vi "myRIO_BRig_FPGA_v2,5__PortC.vi"() -> ()   [LabVIEW 2014]
uses:
  <vilib>/rvi/FXPMathLib/FxpDiv/subVIs/nifxpmath_Div_SimConfig.ctl
  <vilib>/rvi/FXPMathLib/FxpSinAndCos/subVIs/nifxpmath_SinAndCos_SimConfig.ctl
  <vilib>/rvi/FXPMathLib/FxpDiv/simVIs/DllFxpDivTemp_sub.vi
  <vilib>/rvi/FXPMathLib/FxpSinAndCos/simVIs/DllFxpSinAndCosTemp_sub.vi
  <vilib>/rvi/Emulation/niFpgaGetClockAttributes.vi
  <vilib>/rvi/Emulation/niFpgaSctlEmulationGetInTimedLoop.vi
  <vilib>/rvi/Emulation/niFpgaEmulationReportErrorSimple.vi
  <vilib>/rvi/eio/common/nirviEmuTemplateMethod_errors.vi
  <vilib>/rvi/Emulation/niFpgaCriticalErrorInLSC.vi
  <vilib>/rvi/FXPMathLib/FxpDiv/XNode/nifxpmath_Div.xnode
  <vilib>/rvi/FXPMathLib/FxpMul/XNode/nifxpmath_Multiplier.xnode
  <vilib>/rvi/FXPMathLib/FxpSinAndCos/XNode/nifxpmath_SinAndCos.xnode
  <vilib>/rvi/FXPMathLib/FxpSub/XNode/nifxpmath_Sub.xnode
  <vilib>/eio/EIONode/EIONode.xnode
  <vilib>/rvi/FXPMathLib/sim/FxpSim.dll
panel:
  in  "laserledMTrig":bool
  in  "tCycle_laser_wro":u32=100
  in  "tDelay_laser_wro":u32
  in  "tCycle_laser_rew":u32=100
  in  "tDelay_laser_rew":u32
  in  "laserResponse_reward_LED":bool
  in  "laserResponse_wrong_LED":bool
  out "SelectWrong":bool
  out "SelectReward":bool
  in  "laserResponse_wrong":bool
  in  "laserResponse_reward":bool
  in  "Left(F)_or_Right(T)":bool
  in  "ignoreWrong":bool
  in  "SelectionState":bool
  in  "laserMTrig":bool
  in  "FPGA_Stop":bool
  in  "audioTrigger_L":bool
  in  "audioTrigger_R":bool
  in  "audioFreq_L_Hz":u16=1000 min=1000 max=14000 step=1000
  in  "audioAmp_L":u16=1 min=1 max=32767 step=1
  in  "audioFreq_R_Hz":u16=1000 min=1000 max=14000 step=1000
  in  "audioAmp_R":u16=1 min=1 max=32767 step=1
  in  "A3_SL":bool
  in  "A1_SR":bool
  in  "Counts_Reset":bool
  out "A4_LickR":u32
  out "A2_LickL":u32
  in  "A6_Act":bool
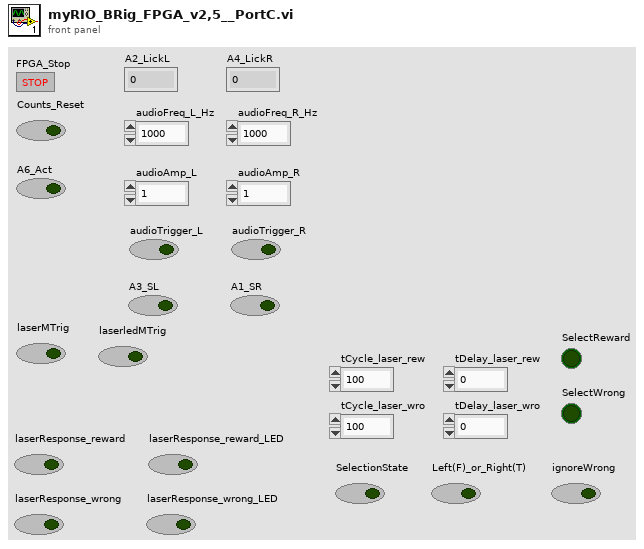
[diagram p1: front panel]
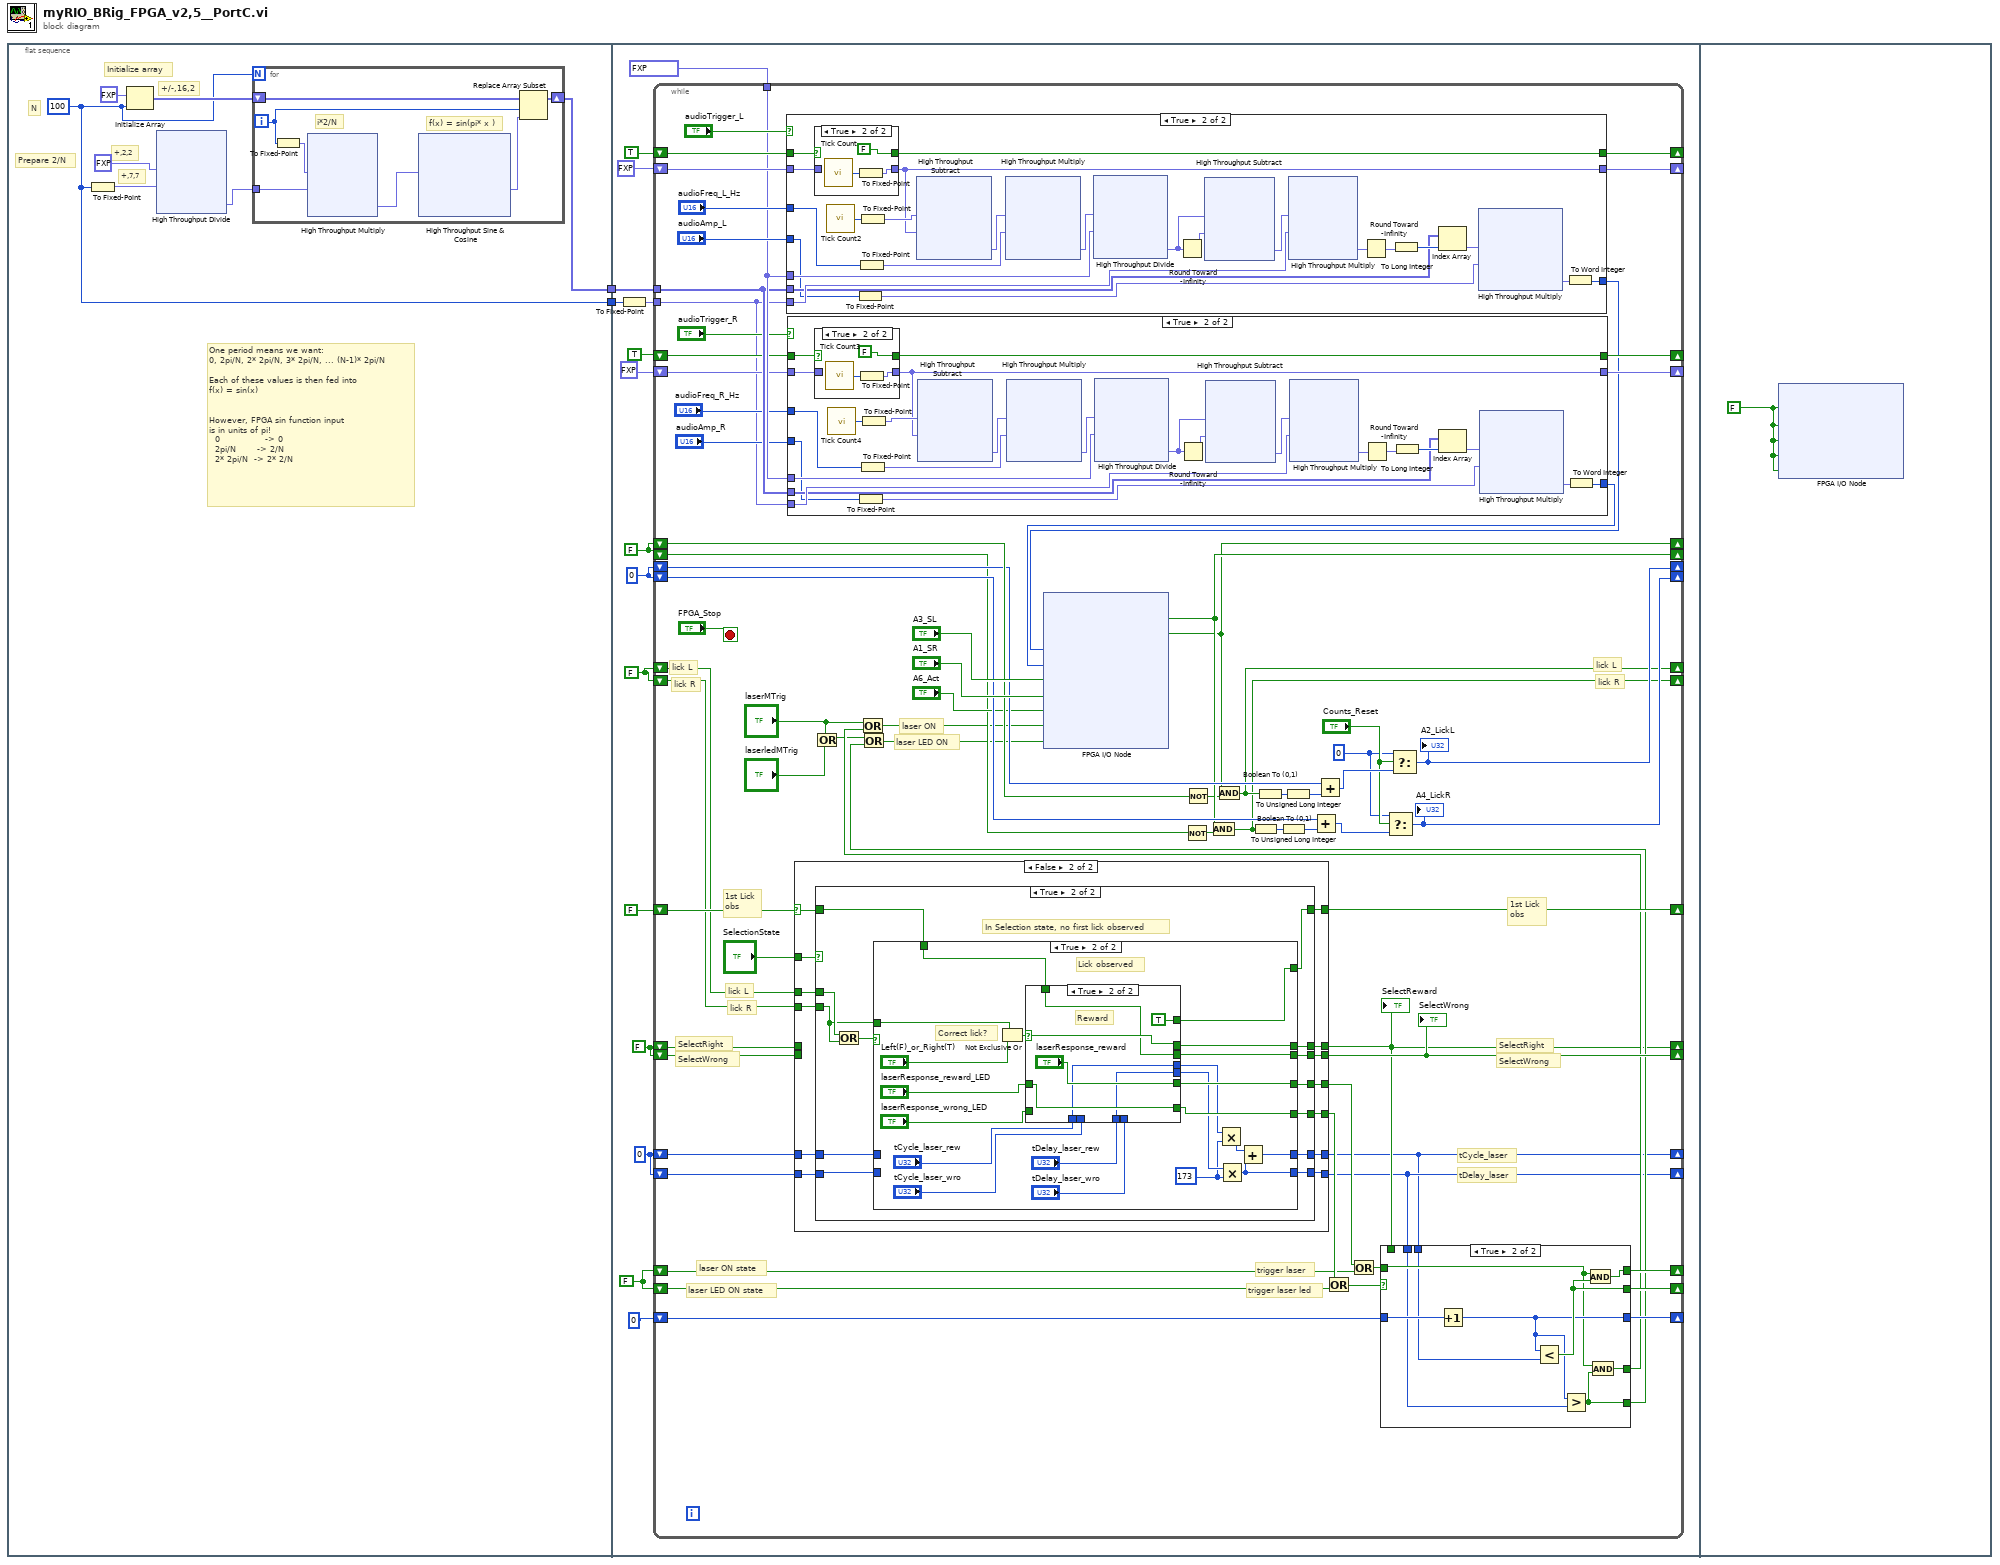
[diagram p0: block diagram]
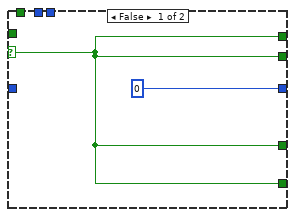
[diagram p2: hidden frame]
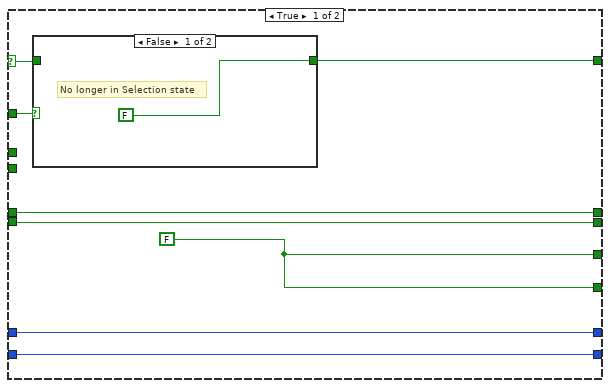
[diagram p3: hidden frame]
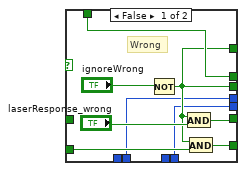
[diagram p7: hidden frame]
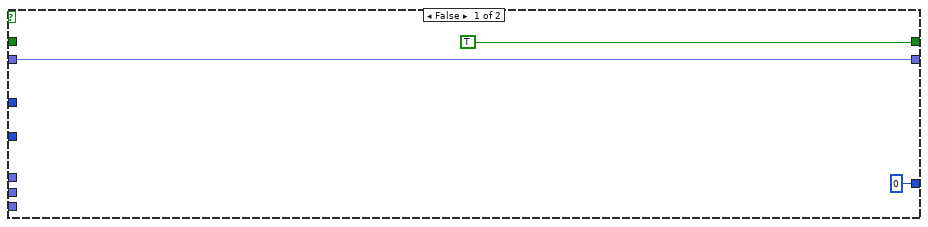
[diagram p8: hidden frame]
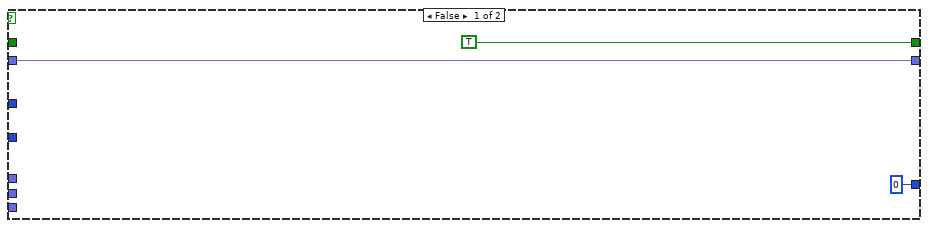
[diagram p10: hidden frame]
diagram:
  n1 = flat-sequence {
    tunnel: [w4] -> w2
    tunnel: [w3] -> w1
    tunnel: w2 -> [w84]
    tunnel: w1 -> [w86]
    frame #0 {
      w3 = 100 ("dimension size")
      # "N"
      # "+,7,7"
      # "+,2,2"
      # "+/-,16,2"
      # "Prepare 2/N"
      # "One period means we want:\n0, 2pi/N, 2* 2pi/N, 3* 2pi/N, ... (N-1)* 2pi/N\n\nEach of these values is then fed into\nf(x) = sin(x)\n\n\nHowever, FPGA sin function input\nis in units of pi!\n  0               -> 0\n  2pi/N       -> 2/N\n  2* 2pi/N  -> 2* 2/N"
      # "Initialize array"
      n2 = To Fixed-Point(number=w3) -> (fixed-point=w6:fxp<+,7,7>)  [unwired: 1 in]
      n3 = Initialize Array(fxp<+/-,16,2> 0.0 ("element"), w3) -> (w9:fxp<+/-,16,2>[])
      n4 = xnode "High Throughput Divide"("x"=fxp<+,2,2> 2.0, "y"=w6) -> ("x/y"=w5:fxp<+,27,0>)
      n5 = for {
        N: w3 -> [_]
        shift-right: [w42] -> w4
        shift-left: w9 -> [w43]
        tunnel: w5 -> [w38]
        i -> [w41]
        # "f(x) = sin(pi* x )"
        # "i*2/N"
        n6 = To Fixed-Point(number=w41) -> (fixed-point=w39:fxp<+,7,7>)  [unwired: 1 in]
        n7 = xnode ("High Throughput Multiply")("x"=w39, "y"=w38) -> ("x*y"=w37:fxp<+,34,7>)
        n8 = xnode "High Throughput Sine & Cosine"("x (pi)"=w37) -> ("sin(x)"=w40:fxp<+/-,16,2>)  [unwired: 1 out]
        n9 = Replace Array Subset(array=w43, new element=w40, index=w41) -> (w42:fxp<+/-,16,2>[])
      }
    }
    frame #1 {
      w74 = u32 0
      w76 = FALSE
      w75 = FALSE
      w79 = FALSE
      w80 = FALSE
      w81 = u32 0
      n10 = To Fixed-Point(number=w86) -> (fixed-point=w85:fxp<+,7,7>)  [unwired: 1 in]
      n11 = while {
        shift-right: [w156] -> _
        shift-left: TRUE -> [w160]
        shift-right: [w155] -> _
        shift-left: fxp<+,32,32> 0.0 -> [w159]
        tunnel: fxp<+,17,26> 40000000.0 -> [w154]
        tunnel: w85 -> [w147]
        tunnel: w84 -> [w153]
        shift-right: [w146] -> _
        shift-left: TRUE -> [w152]
        shift-right: [w145] -> _
        shift-left: fxp<+,32,32> 0.0 -> [w151]
        shift-right: [w122] -> _
        shift-left: w81 -> [w134]
        shift-right: [w125] -> _
        shift-left: w81 -> [w138]
        shift-right: [w126] -> _
        shift-left: w80 -> [w129]
        shift-right: [w123] -> _
        shift-left: w80 -> [w135]
        shift-right: [w120] -> _
        shift-left: FALSE -> [w119]
        shift-right: [w118] -> _
        shift-left: w79 -> [w116]
        shift-right: [w117] -> _
        shift-left: w79 -> [w115]
        shift-right: [w105] -> _
        shift-left: w75 -> [w107]
        shift-right: [w113] -> _
        shift-left: u32 0 -> [w114]
        shift-right: [w97] -> _
        shift-left: w76 -> [w111]
        shift-right: [w112] -> _
        shift-left: w76 -> [w110]
        shift-right: [w106] -> _
        shift-left: w75 -> [w101]
        shift-right: [w93] -> _
        shift-left: w74 -> [w96]
        shift-right: [w94] -> _
        shift-left: w74 -> [w95]
        stop <- "FPGA_Stop" stop-if-true
        w131 = u32 0
        # "tDelay_laser"
        # "tCycle_laser"
        # "laser LED ON"
        # "laser ON"
        # "laser LED ON state"
        # "laser ON state"
        # "SelectWrong"
        # "SelectRight"
        # "SelectWrong"
        # "SelectRight"
        # "lick R"
        # "lick L"
        # "1st Lick\nobs"
        # "1st Lick\nobs"
        # "lick R"
        # "lick L"
        # "lick R"
        # "lick L"
        # "trigger laser led"
        # "trigger laser"
        n12 = case shown="True" "audioTrigger_L" {
          tunnel: w160 -> [_ w338]
          tunnel: w159 -> [w314 w337]
          tunnel: "audioFreq_L_Hz" -> [_ w334]
          tunnel: w154 -> [_ w331]
          tunnel: [w314 w315] -> w155
          tunnel: [TRUE w328] -> w156
          tunnel: w147 -> [_ w327]
          tunnel: w153 -> [_ w322]
          tunnel: "audioAmp_L" -> [_ w320]
          tunnel: [i16 0 w317] -> w141
          frame False {
          }
          frame True {
            n13 = case shown="True" w338 {
              selector: w338 -> [w367 _]
              tunnel: [w367 FALSE] -> w328
              tunnel: w337 -> [w366 _]
              tunnel: [w366 w368] -> w315
              frame False {
              }
              frame True {
                n14 = call "Tick Count"() -> ("Tick Count(Ticks)"=w370:u32)
                n15 = To Fixed-Point(number=w370) -> (fixed-point=w368:fxp<+,32,32>)  [unwired: 1 in]
              }
            }
            n16 = call "Tick Count2"() -> ("Tick Count(Ticks)"=w336:u32)
            n17 = To Fixed-Point(number=w320) -> (fixed-point=w319:fxp<+,15,15>)  [unwired: 1 in]
            n18 = To Fixed-Point(number=w334) -> (fixed-point=w333:fxp<+,14,14>)  [unwired: 1 in]
            n19 = To Fixed-Point(number=w336) -> (fixed-point=w316:fxp<+,32,32>)  [unwired: 1 in]
            n20 = xnode "High Throughput Subtract"("x"=w316, "y"=w315) -> ("x-y"=w335:fxp<+,32,32>)
            n21 = xnode ("High Throughput Multiply")("x"=w335, "y"=w333) -> ("x*y"=w332:fxp<+,46,46>)
            n22 = xnode "High Throughput Divide"("x"=w332, "y"=w331) -> ("x/y"=w330:fxp<+,34,21>)
            n23 = Round Toward -Infinity(1:w330) -> (0:w329:fxp<+,21,21>)
            n24 = xnode "High Throughput Subtract"("x"=w330, "y"=w329) -> ("x-y"=w326:fxp<+,14,1>)
            n25 = xnode ("High Throughput Multiply")("x"=w326, "y"=w327) -> ("x*y"=w323:fxp<+,21,8>)
            n26 = Round Toward -Infinity(1:w323) -> (0:w325:fxp<+,8,8>)
            n27 = To Long Integer(number=w325) -> (32bit integer=w324:i32)
            n28 = Index Array(array=w322, index=w324) -> (element=w321:fxp<+/-,16,2>)
            n29 = xnode ("High Throughput Multiply")("x"=w321, "y"=w319) -> ("x*y"=w318:fxp<+/-,31,17>)
            n30 = To Word Integer(number=w318) -> (16bit integer=w317:i16)
          }
        }
        n31 = case shown="True" "audioTrigger_R" {
          tunnel: w152 -> [_ w279]
          tunnel: w151 -> [w255 w278]
          tunnel: "audioFreq_R_Hz" -> [_ w275]
          tunnel: w154 -> [_ w272]
          tunnel: [w255 w256] -> w145
          tunnel: [TRUE w269] -> w146
          tunnel: w147 -> [_ w268]
          tunnel: w153 -> [_ w263]
          tunnel: "audioAmp_R" -> [_ w261]
          tunnel: [i16 0 w258] -> w142
          frame False {
          }
          frame True {
            n32 = case shown="True" w279 {
              selector: w279 -> [w308 _]
              tunnel: [w308 FALSE] -> w269
              tunnel: w278 -> [w307 _]
              tunnel: [w307 w309] -> w256
              frame False {
              }
              frame True {
                n33 = call "Tick Count3"() -> ("Tick Count(Ticks)"=w311:u32)
                n34 = To Fixed-Point(number=w311) -> (fixed-point=w309:fxp<+,32,32>)  [unwired: 1 in]
              }
            }
            n35 = call "Tick Count4"() -> ("Tick Count(Ticks)"=w277:u32)
            n36 = To Fixed-Point(number=w261) -> (fixed-point=w260:fxp<+,15,15>)  [unwired: 1 in]
            n37 = To Fixed-Point(number=w275) -> (fixed-point=w274:fxp<+,14,14>)  [unwired: 1 in]
            n38 = To Fixed-Point(number=w277) -> (fixed-point=w257:fxp<+,32,32>)  [unwired: 1 in]
            n39 = xnode "High Throughput Subtract"("x"=w257, "y"=w256) -> ("x-y"=w276:fxp<+,32,32>)
            n40 = xnode ("High Throughput Multiply")("x"=w276, "y"=w274) -> ("x*y"=w273:fxp<+,46,46>)
            n41 = xnode "High Throughput Divide"("x"=w273, "y"=w272) -> ("x/y"=w271:fxp<+,34,21>)
            n42 = Round Toward -Infinity(1:w271) -> (0:w270:fxp<+,21,21>)
            n43 = xnode "High Throughput Subtract"("x"=w271, "y"=w270) -> ("x-y"=w267:fxp<+,14,1>)
            n44 = xnode ("High Throughput Multiply")("x"=w267, "y"=w268) -> ("x*y"=w264:fxp<+,21,8>)
            n45 = Round Toward -Infinity(1:w264) -> (0:w266:fxp<+,8,8>)
            n46 = To Long Integer(number=w266) -> (32bit integer=w265:i32)
            n47 = Index Array(array=w263, index=w265) -> (element=w262:fxp<+/-,16,2>)
            n48 = xnode ("High Throughput Multiply")("x"=w262, "y"=w260) -> ("x*y"=w259:fxp<+/-,31,17>)
            n49 = To Word Integer(number=w259) -> (16bit integer=w258:i16)
          }
        }
        n50 = case shown="False" w119 {
          selector: w119 -> [w179 w194]
          tunnel: "SelectionState" -> [w181 w196]
          tunnel: [w180 w195] -> w120
          tunnel: w116 -> [_ w193]
          tunnel: w115 -> [_ w192]
          tunnel: [w178 w191] -> w102
          tunnel: [w176 w190] -> w97
          tunnel: [w177 w189] -> w112
          tunnel: w111 -> [w176 _]
          tunnel: w110 -> [w177 _]
          tunnel: [w178 w188] -> w108
          tunnel: [w175 w187] -> w93
          tunnel: [w174 w186] -> w94
          tunnel: w96 -> [w175 w185]
          tunnel: w95 -> [w174 w184]
          frame True {
            w178 = FALSE
            n51 = case shown="False" w181 {
              tunnel: [FALSE w183] -> w180
              tunnel: w179 -> [_ w183]
              frame False {
                # "No longer in Selection state"
              }
              frame True {
                # "Already observed first lick, no other action"
              }
            }
          }
          frame False {
            n52 = case shown="True" w196 {
              tunnel: [w199 w209] -> w195
              tunnel: w194 -> [w199 w205]
              tunnel: w193 -> [_ w211]
              tunnel: w192 -> [_ w210]
              tunnel: [w199 w208] -> w191
              tunnel: [w199 w207] -> w190
              tunnel: [w199 w206] -> w189
              tunnel: [w199 w204] -> w188
              tunnel: [w198 w203] -> w187
              tunnel: [w197 w202] -> w186
              tunnel: w185 -> [w198 w201]
              tunnel: w184 -> [w197 w200]
              frame False {
                # "Not in Selection state"
              }
              frame True {
                # "In Selection state, no first lick observed"
                n53 = Or(x=w211, y=w210) -> (x .or. y?=w212:bool)
                n54 = case shown="True" w212 {
                  tunnel: w210 -> [_ w235]
                  tunnel: [w215 w228] -> w209
                  tunnel: [w215 w233] -> w208
                  tunnel: [w215 w232] -> w207
                  tunnel: [w215 w231] -> w206
                  tunnel: w205 -> [w215 w230]
                  tunnel: [w215 w229] -> w204
                  tunnel: [w214 w217] -> w203
                  tunnel: [w213 w216] -> w202
                  tunnel: w201 -> [w214 _]
                  tunnel: w200 -> [w213 _]
                  frame False {
                  }
                  frame True {
                    w218 = u32 173
                    # "Correct lick?"
                    # "Lick observed"
                    n55 = Not Exclusive Or(1:"Left(F)_or_Right(T)", 2:w235) -> (0:w234:bool)
                    n56 = case shown="True" w234 {
                      selector: w234 -> [_ w251]
                      tunnel: [w242 "laserResponse_reward"] -> w233
                      tunnel: [w240 w247] -> w231
                      tunnel: [w244 w251] -> w232
                      tunnel: w230 -> [w244 w247]
                      tunnel: [w241 w249] -> w229
                      tunnel: [w240 TRUE] -> w228
                      tunnel: "laserResponse_reward_LED" -> [_ w249]
                      tunnel: "laserResponse_wrong_LED" -> [w239 _]
                      tunnel: "tCycle_laser_rew" -> [_ w246]
                      tunnel: "tCycle_laser_wro" -> [w237 _]
                      tunnel: "tDelay_laser_rew" -> [_ w248]
                      tunnel: "tDelay_laser_wro" -> [w238 _]
                      tunnel: [w238 w248] -> w220
                      tunnel: [w237 w246] -> w219
                      frame False {
                        # "Wrong"
                        n57 = Not(x="ignoreWrong") -> (.not. x?=w240:bool)
                        n58 = And(x=w240, y="laserResponse_wrong") -> (x .and. y?=w242:bool)
                        n59 = And(x=w240, y=w239) -> (x .and. y?=w241:bool)
                      }
                      frame True {
                        # "Reward"
                      }
                    }
                    n60 = Multiply(x=w219, y=w218) -> (x*y=w221:u32)
                    n61 = Multiply(x=w220, y=w218) -> (x*y=w216:u32)
                    n62 = Add(x=w221, y=w216) -> (x+y=w217:u32)
                  }
                }
              }
            }
          }
        }
        "SelectWrong" <- w112
        "SelectReward" <- w97
        n63 = Or(x="laserMTrig", y="laserledMTrig") -> (x .or. y?=w91:bool)
        n64 = Not(x=w129) -> (.not. x?=w128:bool)
        n65 = Not(x=w135) -> (.not. x?=w124:bool)
        n66 = Or(x=w108, y=w107) -> (x .or. y?=w109:bool)
        n67 = Or(x=w102, y=w101) -> (x .or. y?=w100:bool)
        n68 = case shown="True" w109 {
          selector: w109 -> [w163 _]
          tunnel: w114 -> [_ w173]
          tunnel: [u32 0 w170] -> w113
          tunnel: [w163 w171] -> w105
          tunnel: [w163 w172] -> w106
          tunnel: w100 -> [_ w169]
          tunnel: [w163 w168] -> w98
          tunnel: [w163 w167] -> w99
          tunnel: w97 -> [_ _]
          tunnel: w94 -> [_ w166]
          tunnel: w93 -> [_ w165]
          frame False {
          }
          frame True {
            n69 = Increment(x=w173) -> (x+1=w170:u32)
            n70 = Less?(x=w170, y=w165) -> (x < y?=w171:bool)
            n71 = Greater?(x=w170, y=w166) -> (0:w168:bool)
            n72 = And(x=w169, y=w171) -> (x .and. y?=w172:bool)
            n73 = And(x=w169, y=w168) -> (x .and. y?=w167:bool)
          }
        }
        n74 = Or(x="laserMTrig", y=w99) -> (x .or. y?=w104:bool)
        n75 = Or(x=w91, y=w98) -> (x .or. y?=w103:bool)
        n76 = xnode "FPGA I/O Node"("AudioOut/Left"=w141, "AudioOut/Right"=w142, "ConnectorC/DIO3"="A3_SL", "ConnectorC/DIO1"="A1_SR", "ConnectorC/DIO6"="A6_Act", "ConnectorC/DIO0"=w104, "ConnectorC/DIO7"=w103) -> ("ConnectorC/DIO4"=w126:bool, "ConnectorC/DIO2"=w123:bool)  [unwired: 9 in, 9 out]
        n77 = And(x=w126, y=w128) -> (x .and. y?=w117:bool)
        n78 = And(x=w123, y=w124) -> (x .and. y?=w118:bool)
        n79 = Boolean To (0,1)(Boolean=w117) -> (0, 1=w140:i16)
        n80 = Boolean To (0,1)(Boolean=w118) -> (0, 1=w137:i16)
        n81 = To Unsigned Long Integer(number=w140) -> (unsigned 32bit integer=w139:u32)
        n82 = To Unsigned Long Integer(number=w137) -> (unsigned 32bit integer=w136:u32)
        n83 = Add(x=w138, y=w139) -> (x+y=w127:u32)
        n84 = Add(x=w134, y=w136) -> (x+y=w133:u32)
        n85 = Select(t=w131, s="Counts_Reset", f=w127) -> (s? t:f=w125:u32)
        "A4_LickR" <- w125
        n86 = Select(t=w131, s="Counts_Reset", f=w133) -> (s? t:f=w122:u32)
        "A2_LickL" <- w122
      }
    }
    frame #2 {
      w371 = FALSE ("ConnectorA/DIO3")
      n87 = xnode "FPGA I/O Node"("ConnectorC/DIO3"=w371, "ConnectorC/DIO1"=w371, "ConnectorC/DIO0"=w371, "ConnectorC/DIO6"=w371, "ConnectorC/DIO7"=w371) -> ()  [unwired: 5 in, 5 out]
    }
  }
